vi "Conveyor and Shooter SS Controls to Commands 2017.vi"(11 "Pilot-CoPilot Controls":T2) -> (3 "Shooter and Conveyor Commands":T1)   [LabVIEW 2016]
uses:
  Robot Control Outputs 2017.ctl
  Conveyor and Shooter Commands.ctl
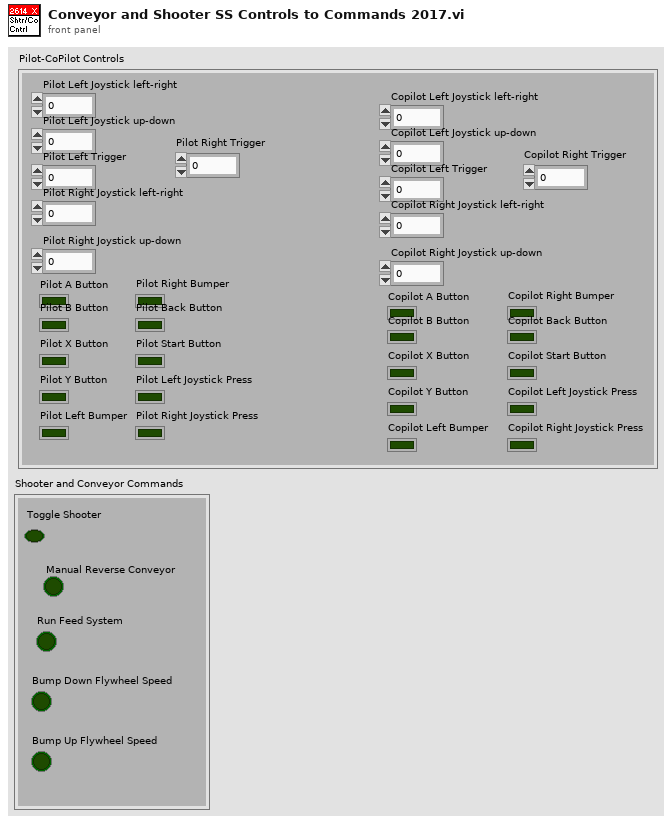
[diagram p1: front panel]
types:
  T1 = typedef "Conveyor and Shooter Commands.ctl" = cluster{"Toggle Shooter":bool, "Manual Reverse Conveyor":bool, "Run Feed System":bool, "Bump Down Flywheel Speed":bool, "Bump Up Flywheel Speed":bool}
  T2 = typedef "Robot Control Outputs 2017.ctl" = cluster{"Pilot Left Joystick left-right":dbl, "Pilot Left Joystick up-down":dbl, "Pilot A Button":bool, "Pilot B Button":bool, "Pilot X Button":bool, "Pilot Y Button":bool, "Pilot Left Bumper":bool, "Pilot Right Bumper":bool, "Pilot Back Button":bool, "Pilot Start Button":bool, "Pilot Left Joystick Press":bool, "Pilot Right Joystick Press":bool, "Pilot Left Trigger":dbl, "Pilot Right Joystick left-right":dbl, "Pilot Right Joystick up-down":dbl, "Pilot Right Trigger":dbl, "Copilot Left Joystick left-right":dbl, "Copilot Left Joystick up-down":dbl, "Copilot A Button":bool, "Copilot B Button":bool, "Copilot X Button":bool, "Copilot Y Button":bool, "Copilot Left Bumper":bool, "Copilot Right Bumper":bool, "Copilot Back Button":bool, "Copilot Start Button":bool, "Copilot Left Joystick Press":bool, "Copilot Right Joystick Press":bool, "Copilot Left Trigger":dbl, "Copilot Right Joystick left-right":dbl, "Copilot Right Joystick up-down":dbl, "Copilot Right Trigger":dbl}
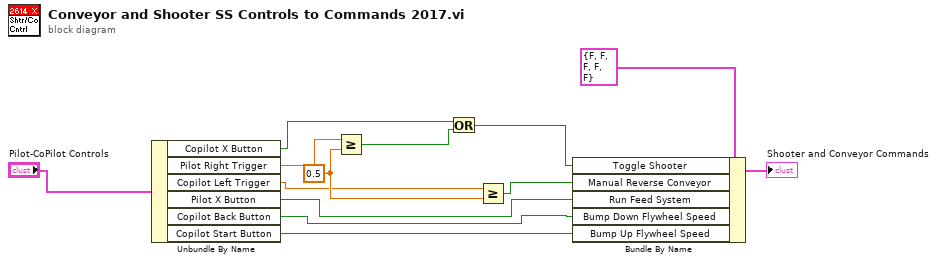
[diagram p0: block diagram]
diagram:
  w9 = 0.5 ("y")
  n1 = Unbundle By Name("Pilot-CoPilot Controls") -> ("Copilot X Button"=w1:bool, "Pilot Right Trigger"=w10:dbl, "Copilot Left Trigger"=w8:dbl, "Pilot X Button"=w6:bool, "Copilot Back Button"=w5:bool, "Copilot Start Button"=w4:bool)
  n2 = Greater Or Equal?(x=w10, y=w9) -> (x >= y?=w3:bool)
  n3 = Or(x=w1, y=w3) -> (x .or. y?=w2:bool)
  n4 = Greater Or Equal?(x=w8, y=w9) -> (x >= y?=w7:bool)
  n5 = Bundle By Name(cluster=T1 {"Toggle Shooter"=FALSE, "Manual Reverse Conveyor"=FALSE, "Run Feed System"=FALSE, "Bump Down Flywheel Speed"=FALSE, "Bump Up Flywheel Speed"=FALSE} ("Shooter and Conveyor Commands"), "Toggle Shooter"=w2, "Manual Reverse Conveyor"=w7, "Run Feed System"=w6, "Bump Down Flywheel Speed"=w5, "Bump Up Flywheel Speed"=w4) -> (→"Shooter and Conveyor Commands":T1)
